vi "qREC DAT to Array.vi"(0 "System no.":i32=1 min=1 max=4 step=1, 1 "RecorderID":string, 2 "RecorderFormat":string="ASCII", 3 "StartPoint":i32 min=1 max=4 step=1, 4 "NumberOfPoints":i32 min=1 max=4 step=1, 5 "error in":errorcluster, 7 "TraceID":i32 min=1 max=4 step=1) -> (14 "GCSArray Header":T1={"Identifier"="", "Version"=0, "Remark"="", "Dimension"=0, "Type"=enum."Matrix", "Separator"=0, "NData"=0, "NData%"=[], "Name%"=[], "Start%"=[], "End%"=[], "Delta%"=[], "SampleTime"=inf, "TransmittedUnit%"=[], "DisplayedUnit%"=[], "RatioNominator%"=[], "RatioDenominator%"=[]}, 15 "GCSArray data":dbl[][](array[numeric]), 19 "error out":errorcluster)   [LabVIEW 2020]
doc: "Get Recorder Data Values.\n\nThis VI reads the data recorder and returns a LabVIEW compatible data description."
uses:
  Support/GCSArray_header.ctl
  Support/GCSArray_regex_range.ctl
panel:
  # "Get Recorded Data Values."
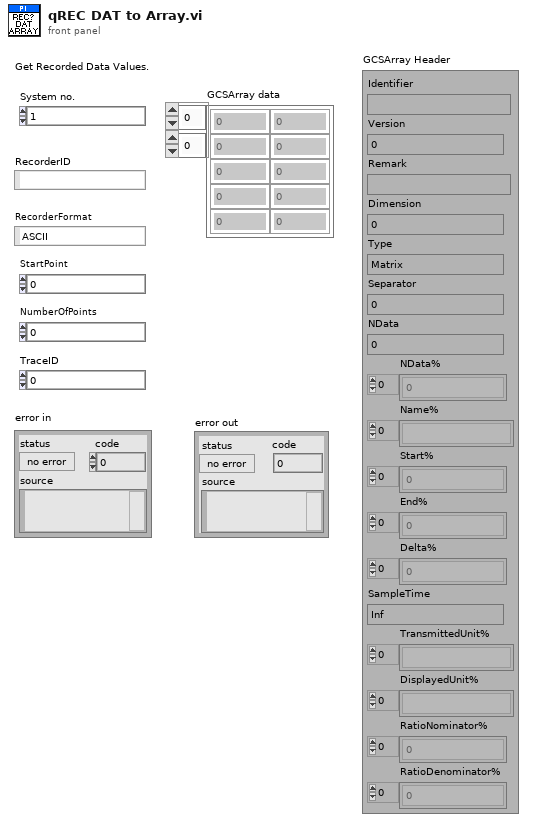
[diagram p1: front panel]
types:
  T1 = typedef "GCSArray_header.ctl" = cluster{"Identifier":string, "Version":i32, "Remark":string, "Dimension":i32, "Type":enum16{"Matrix", "Table"}, "Separator":u8, "NData":i32, "NData%":i32[], "Name%":string[], "Start%":dbl[], "End%":dbl[], "Delta%":dbl[], "SampleTime":dbl, "TransmittedUnit%":string[], "DisplayedUnit%":string[], "RatioNominator%":dbl[], "RatioDenominator%":dbl[]}
  T2 = typedef "GCSArray_regex_range.ctl" = cluster{"Begin":i32, "End":i32}
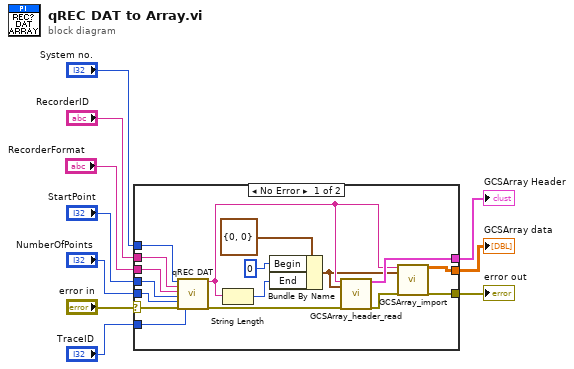
[diagram p0: block diagram]
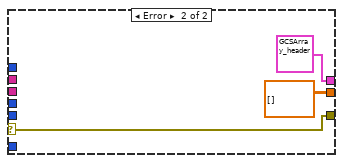
[diagram p2: hidden frame]
diagram:
  n1 = case shown="No Error" "error in" {
    selector: "error in" -> [w26 w30]
    tunnel: [w20 w30] -> w9
    tunnel: "NumberOfPoints" -> [w22 _]
    tunnel: "StartPoint" -> [w23 _]
    tunnel: "TraceID" -> [w21 _]
    tunnel: "System no." -> [w27 _]
    tunnel: "RecorderID" -> [w25 _]
    tunnel: "RecorderFormat" -> [w24 _]
    tunnel: [w19 dbl[][] [] ("GCSArray data")] -> w2
    tunnel: [w18 T1 {"Identifier"="", "Version"=0, "Remark"="", "Dimension"=0, "Type"=enum."Matrix", "Separator"=0, "NData"=0, "NData%"=[], "Name%"=[], "Start%"=[], "End%"=[], "Delta%"=[], "SampleTime"=inf, "TransmittedUnit%"=[], "DisplayedUnit%"=[], "RatioNominator%"=[], "RatioDenominator%"=[]} ("GCSArray Header")] -> w1
    frame No Error {
      n2 = call "qREC DAT.vi"("System no."=w27, "RecorderID"=w25, "RecorderFormat"=w24, "StartPoint"=w23, "NumberOfPoints"=w22, "error in"=w26, "TraceID"=w21) -> ("Recorded data as GCSArray"=w13:string, "error out"=w16:errorcluster)  [unwired: 11 in]
      n3 = String Length(string=w13) -> (length=w12:i32)
      n4 = Bundle By Name(cluster=T2 {"Begin"=0, "End"=0} ("Range"), "Begin"=0, "End"=w12) -> (w11:T2)
      n5 = call "GCSArray_header_read.vi"("GCSArray input string"=w13, "Range"=w11, "error in (no error)"=w16) -> ("GCSArray Header"=w18:T1, "error out"=w17:errorcluster)  [unwired: 15 in]
      n6 = call "GCSArray_import.vi"("GCSArray input string"=w13, "Range"=w11, "error in (no error)"=w17) -> ("GCSArray data"=w19:dbl[][], "error out"=w20:errorcluster)  [unwired: 15 in]
    }
    frame Error {
    }
  }
  "error out" <- w9
  "GCSArray data" <- w2
  "GCSArray Header" <- w1
